vi "Test View No Process Errors Showing and Hiding Panel.vi"(8 "error in (no error)":errorcluster, 11 "UI View Test In":refnum<class "View Test.lvclass">) -> (0 "error out":errorcluster, 3 "UI View Test Out":refnum<class "View Test.lvclass">)   [LabVIEW 2020, in "View Test.lvclass"]
uses:
  View Test.lvclass
  C:/Program Files (x86)/National Instruments/LabVIEW 2020/vi.lib/Asteme/LUnit/Test Case.lvclass
  Framework/Process/Process.lvclass/Process.ctl
  Framework/View/View.lvclass/View.ctl
  <vilib>/Asteme/LUnit/Test Case.lvclass/Test Case.ctl
  <vilib>/Asteme/LUnit/LUnit Assertion Result.lvclass/LUnit Assertion Result.ctl
  Framework/Process/Protected/SubVIs/Get Access Mode.vi
  Framework/View/Public/Get View VI Reference.vi
  Framework/Process/Protected/Messaging/Enqueue Message.vi
  <vilib>/Asteme/LUnit/Palette/Pass.vi
  <vilib>/Asteme/LUnit/Palette/Fail.vi
  <vilib>/Asteme/LUnit/Set Assertion Type.vi
  <vilib>/Utility/error.llb/Clear Errors.vi
  <vilib>/Asteme/LUnit/Variant to string.vi
  Framework/Process/Private/SubVIs/Wait for finish.vi
  Framework/Process/Private/SubVIs/Set Lifecycle State.vi
  Framework/Process/Protected/Messaging/Request Message.vi
  <vilib>/Asteme/LUnit/Add test result.vi
  <vilib>/Asteme/LUnit/LUnit Write Passed.vi
  <vilib>/Asteme/LUnit/LUnit Get Test Case.vi
  <vilib>/Asteme/LUnit/LUnit Write Message.vi
  <vilib>/Asteme/LUnit/LUnit Write Description.vi
  <vilib>/Asteme/LUnit/LUnit Write Assertion Type.vi
  Framework/Process/Private/SubVIs/Enqueue Request Message.vi
  <vilib>/Asteme/LUnit/Read Test Case Name.vi
  Framework/View/View.lvclass
  C:/Users/anton/Documents/GitHub/Triarc-Framework/source/Framework/Process/Process.lvclass
  <vilib>/Utility/error.llb/Error Cluster From Error Code.vi
  Framework/Process/Private/SubVIs/Wait for Response Message.vi
  <vilib>/Asteme/LUnit/Assertion Result/LUnit Get Test Name.vi
  <vilib>/Utility/Data Type/Get Type Information.vi
  <vilib>/Utility/LVClass/Get LV Class Name.vi
  <vilib>/Asteme/LUnit/LUnit Assertion Result.lvclass
  Framework/Process/Process.lvclass
  <vilib>/Asteme/LUnit/Test Case.lvclass
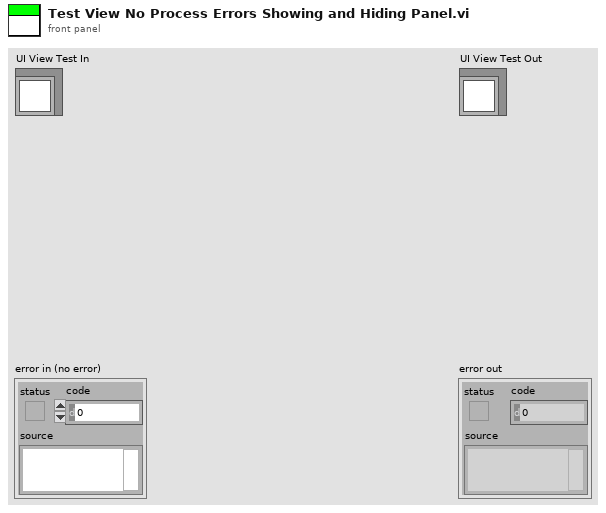
[diagram p1: front panel]
types:
  T1 = typedef "Process.lvclass/Lifecycle State.ctl" = enum16{"Uninitialized", "Initialized", "Started", "Running", "Stopped", "Finished"}
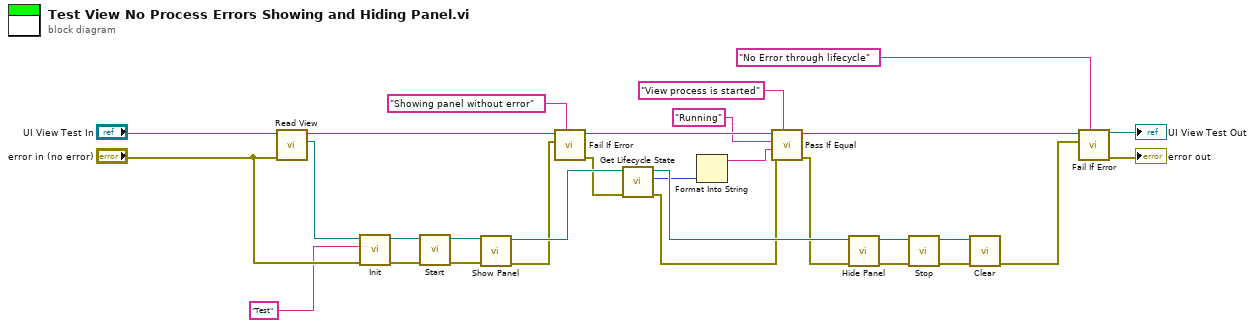
[diagram p0: block diagram]
diagram:
  n1 = call "Read View.vi"("error in (no error)"="error in (no error)", "View Test In"="UI View Test In") -> ("View"=w16:refnum<class "View.lvclass">, "View Test Out"=w27:refnum<class "View Test.lvclass">)  [unwired: 7 in, 1 out]
  n2 = call-dynamic "Init.vi"("error in (no error)"="error in (no error)", "Name"="Test", "View In"=w16) -> ("error out"=w4:errorcluster, "View Out"=w24:refnum<class "View.lvclass">)  [unwired: 7 in]
  n3 = call "Start.vi"("error in (no error)"=w4, "Process In"=w24) -> ("error out"=w5:errorcluster, "Process Out"=w6:refnum<class "View.lvclass">)  [unwired: 8 in]
  n4 = call "Show Panel.vi"("error in (no error)"=w5, "View In"=w6) -> ("error out"=w18:errorcluster, "View Out"=w23:refnum<class "View.lvclass">)  [unwired: 8 in]
  n5 = call <vilib>:"Fail If Error.vi"("Description"="Showing panel without error", "Assert error"=w18, "Test Case In"=w27) -> ("error out"=w13:errorcluster, "Test Case Out"=w19:refnum<class "View Test.lvclass">)  [unwired: 7 in]
  n6 = call "Get Lifecycle State.vi"("error in (no error)"=w13, "Process In"=w23) -> ("error out"=w8:errorcluster, "Lifecycle State"=w12:T1, "Process Out"=w15:refnum<class "View.lvclass">)  [unwired: 6 in, 1 out]
  n7 = Format Into String(w12) -> (resulting string=w11:string)  [unwired: 3 in, 1 out]
  n8 = call <vilib>:"Pass If Equal.vi"("Description"="View process is started", "error in (no error)"=w8, "Actual"=w11, "Expected"="Running", "Test Case In"=w19) -> ("error out"=w7:errorcluster, "Test Case Out"=w14:refnum<class "View Test.lvclass">)  [unwired: 5 in]
  n9 = call "Hide Panel.vi"("error in (no error)"=w7, "View In"=w15) -> ("error out"=w2:errorcluster, "View Out"=w20:refnum<class "View.lvclass">)  [unwired: 8 in]
  n10 = call "Stop.vi"("error in (no error)"=w2, "Process In"=w20) -> ("error out"=w1:errorcluster, "Process Out"=w3:refnum<class "View.lvclass">)  [unwired: 7 in, 1 out]
  n11 = call-dynamic "Clear.vi"("error in (no error)"=w1, "View In"=w3) -> ("error out"=w21:errorcluster)  [unwired: 8 in, 1 out]
  n12 = call <vilib>:"Fail If Error.vi"("Description"="No Error through lifecycle", "Assert error"=w21, "Test Case In"=w14) -> ("error out"=→"error out":errorcluster, "Test Case Out"=→"UI View Test Out":refnum<class "View Test.lvclass">)  [unwired: 7 in]
